vi "Unsubscribe.vi"(7 "Close if last?":bool, 8 "error in (no error)":errorcluster, 10 "Receivers Enqueuer":refnum<class "Message Enqueuer.lvclass">, 11 "AF MQTT Message Channel in":refnum<class "AF MQTT Message Channel.lvclass">) -> (0 "error out":errorcluster, 3 "AF MQTT Message Channel out":refnum<class "AF MQTT Message Channel.lvclass">)   [LabVIEW 2020]
uses:
  AF MQTT Message Channel.lvclass
  <vilib>/ActorFramework/Message Enqueuer/Message Enqueuer.lvclass
  Actor Pub Sub Channels/Pub Sub Message Channel/Pub Sub Message Channel.lvclass
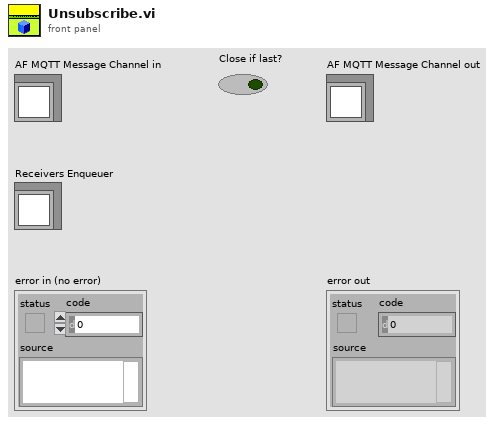
[diagram p1: front panel]
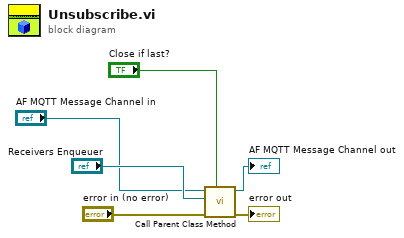
[diagram p0: block diagram]
diagram:
  n1 = call-parent "Call Parent Class Method"("Close if last?"="Close if last?", "error in (no error)"="error in (no error)", "Receivers Enqueuer"="Receivers Enqueuer", "Pub Sub Message Channel in"="AF MQTT Message Channel in") -> ("error out"=→"error out":errorcluster, "Pub Sub Message Channel out"=→"AF MQTT Message Channel out":refnum<class "AF MQTT Message Channel.lvclass">)  [unwired: 6 in]
